vi "SaveFile.vi"(7 "Threshold Exceeded?":bool, 8 "error in (no error)":errorcluster, 9 "sound format":T2, 10 "Filtered Data":waveform(dbl)[](array[waveform]), 11 "sound file refnum in":T1) -> (0 "error out":errorcluster, 3 "sound file refnum out":T1)   [LabVIEW 2019]
uses:
  <vilib>/sound2/lvsound2.llb/Sound File Refnum.ctl
  <vilib>/sound2/lvsound2.llb/Sound File Write Open.vi
  <vilib>/sound2/lvsound2.llb/Sound File Write (DBL).vi
  <vilib>/sound2/lvsound2.llb/Sound Data Format.ctl
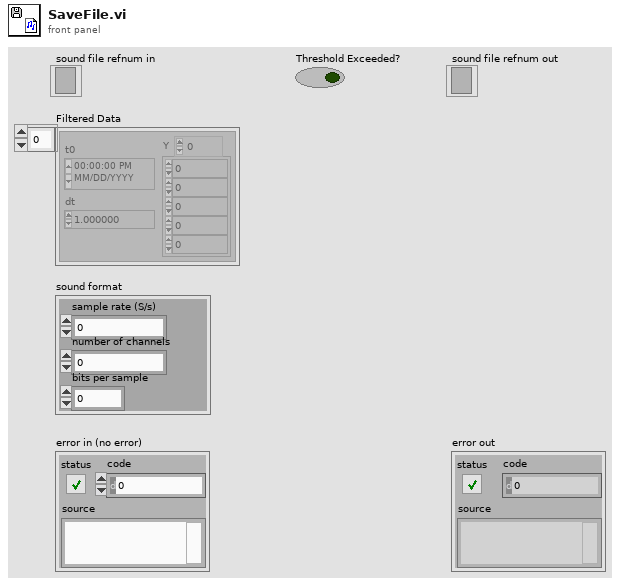
[diagram p1: front panel]
types:
  T1 = typedef "Sound File Refnum.ctl" = refnum<file>
  T2 = typedef "Sound Data Format.ctl" = cluster{"sample rate (S/s)":dbl, "number of channels":i32, "bits per sample":i32}
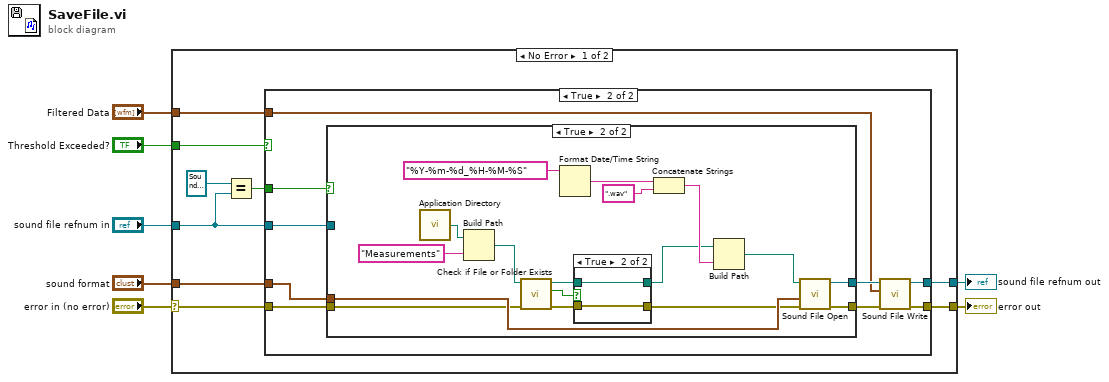
[diagram p0: block diagram]
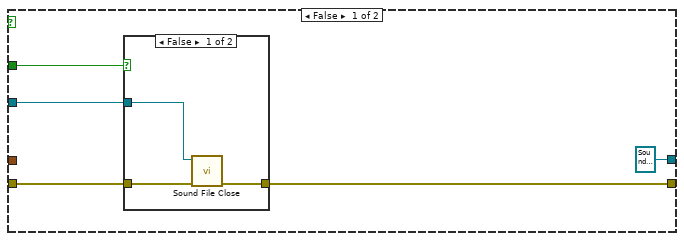
[diagram p2: hidden frame]
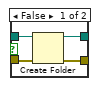
[diagram p5: hidden frame]
diagram:
  n1 = case shown="No Error" "error in (no error)" {
    selector: "error in (no error)" -> [w8 w61]
    tunnel: "Threshold Exceeded?" -> [w16 _]
    tunnel: "Filtered Data" -> [w15 _]
    tunnel: "sound format" -> [w14 _]
    tunnel: [w13 w61] -> w4
    tunnel: [w12 w60] -> w3
    tunnel: "sound file refnum in" -> [w10 w60]
    frame No Error {
      n2 = Equal?(x=T1 refnum ("sound file refnum out"), y=w10) -> (x = y?=w9:bool)
      n3 = case shown="True" w16 {
        tunnel: [w19 w32] -> w13
        tunnel: w14 -> [_ w31]
        tunnel: w15 -> [_ w30]
        tunnel: w8 -> [w21 w29]
        tunnel: [T1 refnum ("sound file refnum out") w28] -> w12
        tunnel: w10 -> [w20 w26]
        tunnel: w9 -> [w17 w27]
        frame False {
          n4 = case shown="False" w17 {
            tunnel: w21 -> [w24 w25]
            tunnel: w20 -> [w23 _]
            tunnel: [w22 w25] -> w19
            frame False {
              n5 = call <vilib>:"Sound File Close.vi"("error in (no error)"=w24, "sound file refnum"=w23) -> ("error out"=w22:errorcluster)  [unwired: 9 in]
            }
            frame True {
            }
          }
        }
        frame True {
          n6 = case shown="True" w27 {
            tunnel: [w35 w53] -> w34
            tunnel: [w36 w52] -> w33
            tunnel: w31 -> [_ w51]
            tunnel: w29 -> [w36 w43]
            tunnel: w26 -> [w35 _]
            frame False {
            }
            frame True {
              n7 = call <vilib>:"Application Directory.vi"() -> ("Application Directory"=w48:path)
              n8 = Build Path(base path=w48, name or relative path="Measurements") -> (appended path=w38:path)
              n9 = call <vilib>:"Check if File or Folder Exists.vi"("error in (no error)"=w43, "path"=w38) -> ("error out"=w42:errorcluster, "file or folder exists?"=w40:bool, "dup path"=w39:path)  [unwired: 7 in]
              n10 = Format Date/Time String(time format string (%c)="%Y-%m-%d_%H-%M-%S") -> (date/time string=w49:string)  [unwired: 2 in]
              n11 = case shown="True" w40 {
                tunnel: w42 -> [w57 w59]
                tunnel: [w56 w59] -> w41
                tunnel: w39 -> [w55 w58]
                tunnel: [w54 w58] -> w37
                frame False {
                  n12 = Create Folder(path (use dialog)=w55, error in=w57) -> (created path=w54:path, error out=w56:errorcluster)  [unwired: 1 in, 1 out]
                }
                frame True {
                }
              }
              n13 = Concatenate Strings(w49, ".wav" ("string")) -> (w50:string)
              n14 = Build Path(base path=w37, name or relative path=w50) -> (appended path=w44:path)
              n15 = call-poly <vilib>:"Sound File Open.vi"("error in (no error)"=w41, "sound format"=w51, "path"=w44) -> ("error out"=w52:errorcluster, "sound file refnum"=w53:T1)  [unwired: 7 in]
            }
          }
          n16 = call-poly <vilib>:"Sound File Write.vi"("error in (no error)"=w33, "data"=w30, "sound file refnum"=w34) -> ("error out"=w32:errorcluster, "sound file refnum out"=w28:T1)  [unwired: 7 in]
        }
      }
    }
    frame Error {
    }
  }
  "error out" <- w4
  "sound file refnum out" <- w3
